vi "DB Path.vi"() -> (3 "DB Path":path)   [LabVIEW 2020, in "SQLITE Inventory.lvlib"]
doc: "Returnd the SataBase path in the application."
uses:
  SQLITE Inventory.lvlib
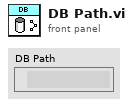
[diagram p1: front panel]
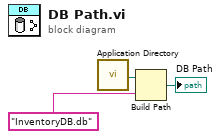
[diagram p0: block diagram]
diagram:
  n1 = call <vilib>:"Application Directory.vi"() -> ("Application Directory"=w2:path)
  n2 = Build Path(base path=w2, name or relative path="InventoryDB.db") -> (appended path=→"DB Path":path)
